vi "Check Status.vi"(8 "error in (no error)":errorcluster, 11 "Photon Counter SR400 in":refnum<class "Photon Counter SR400.lvclass">) -> (0 "error out":errorcluster, 1 "response":string caption="Status", 2 "Ready?":bool, 3 "Photon Counter SR400 out":refnum<class "Photon Counter SR400.lvclass">)   [LabVIEW 2012, in "Photon Counter SR400.lvclass"]
doc: "Checks if the instrument is powered on and updates its member data with the instrument's current status.\n\nNote: it's impossible to get the \"trigger frequency\" (one of the member data) from the instrument itself. Perhaps it shouldn't be part of the member data, but having it as member data makes it possible to give a counting time, which seems like a very important instrumental parameter. Therefore this VI tries to pull the trigger frequency off the existing member data, which won't work when first initialized. Don't know if there will be issues that arise because of that."
uses:
  Photon Counter SR400.lvclass
  Utility Classes/Readable/Readable.lvclass
  Photon Counter SR400.lvclass/Photon Counter SR400.ctl
  SR400/SR400.lvlib
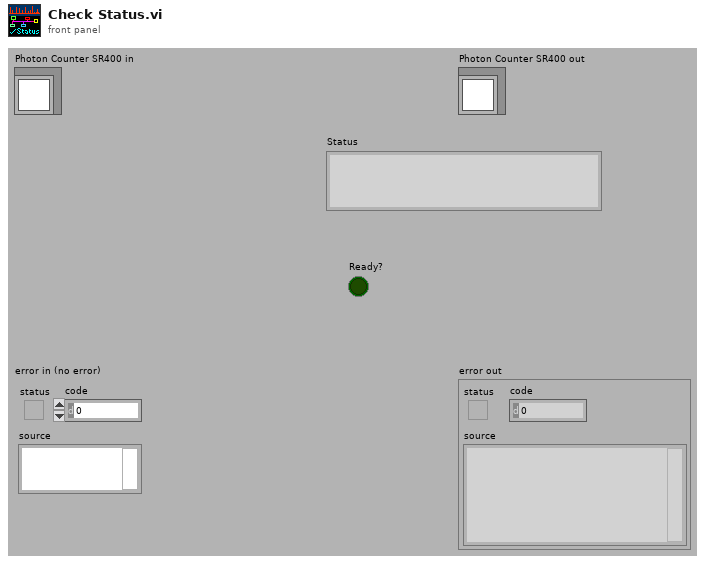
[diagram p1: front panel]
types:
  T1 = typedef "SR400.lvlib/Counter Mode.ctl" = enum16{"A,B For T Preset", "A-B For T Preset", "A+B For T Preset", "A For B Preset"}
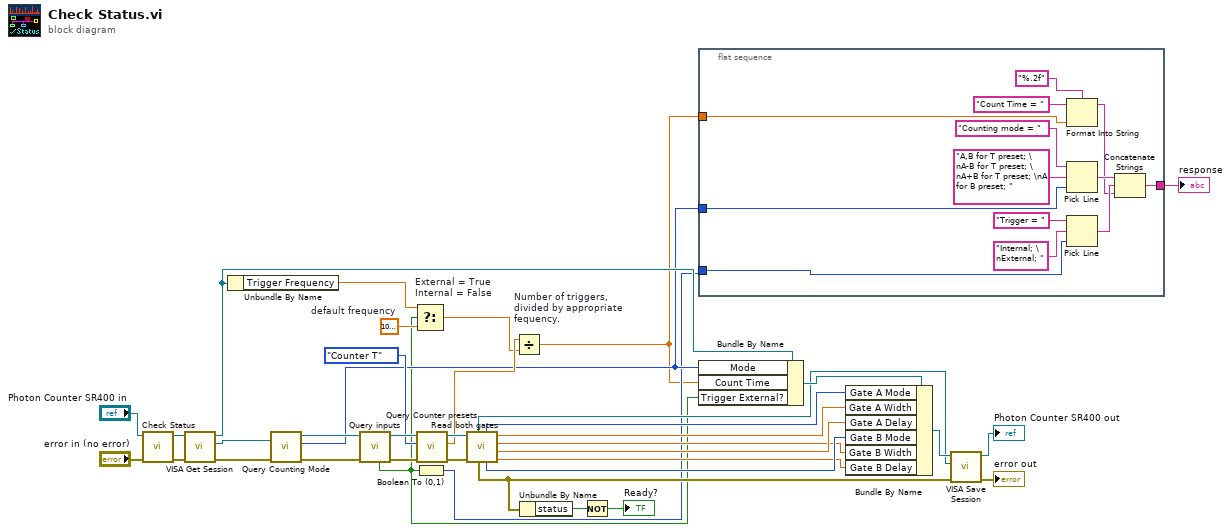
[diagram p0: block diagram]
diagram:
  w9 = dbl[unit] 10000000.0  # default frequency
  n1 = call-parent "Check Status.vi"("error in (no error)"="error in (no error)", "Instrument in"="Photon Counter SR400 in") -> ("error out"=w31:errorcluster, "Instrument out"=w33:refnum<class "Photon Counter SR400.lvclass">)  [unwired: 8 out]
  n2 = call-dynamic "VISA Get Session.vi"("error in (no error)"=w31, "Instrument.lvclass in"=w33) -> ("error out"=w11:errorcluster, "VISA Resource Name"=w1:refnum<visa-resource-name>, "Instrument.lvclass out"=w13:refnum<class "Photon Counter SR400.lvclass">)  [unwired: 7 out]
  n3 = Unbundle By Name(w13) -> ("Trigger Frequency"=w8:dbl[unit])
  n4 = call "Query Counting Mode.vi"("error in (no error)"=w11, "VISA resource name"=w1) -> ("error out"=w10:errorcluster, "output"=w5:T1, "VISA resource name out"=w12:refnum<visa-resource-name>)  [unwired: 7 out]
  n5 = call "Query inputs.vi"("error in (no error)"=w10, "VISA resource name"=w12) -> ("error out"=w25:errorcluster, "VISA resource name out"=w26:refnum<visa-resource-name>, "Externally-triggered?"=w4:bool)  [unwired: 7 out]
  n6 = Select "External = True\nInternal = False"(t=w8, s=w4, f=w9) -> (s? t:f=w6:dbl[unit])
  n7 = Boolean To (0,1)(Boolean=w4) -> (0, 1=w3:i16)
  n8 = call "Query Counter presets.vi"("error in (no error)"=w25, "Counter (Def: T)"=enum16{"Invalid", "Counter B", "Counter T"}."Counter T" ("i (0)"), "VISA resource name"=w26) -> ("error out"=w28:errorcluster, "Number of triggers"=w7:dbl, "VISA resource name out"=w29:refnum<visa-resource-name>)  [unwired: 6 out]
  n9 = call "Read both gates.vi"("error in (no error)"=w28, "VISA resource name"=w29) -> ("Gate B Delay"=w18:dbl[unit], "Gate A Delay"=w21:dbl[unit], "Gate B Width"=w19:dbl[unit], "Gate A Width"=w22:dbl[unit], "Current mode B"=w20:enum16{"CW", "Fixed", "Scan"}, "Current mode A"=w23:enum16{"CW", "Fixed", "Scan"}, "error out"=w15:errorcluster, "VISA resource name out"=w16:refnum<visa-resource-name>)  [unwired: 2 out]
  n10 = Divide "Number of triggers,\ndivided by appropriate\nfequency."(x=w7, y=w6) -> (x/y=w2:dbl[unit])
  n11 = Unbundle By Name(w15) -> ("status"=w14:bool)
  n12 = Not(x=w14) -> (.not. x?=→"Ready?":bool)
  n13 = flat-sequence {
    tunnel: [w46] -> w34
    tunnel: w5 -> [w48]
    tunnel: w3 -> [w43]
    tunnel: w2 -> [w40]
    frame #0 {
      n14 = Format Into String(format string="%.2f", initial string="Count Time = " ("string (\"\")"), w40) -> (resulting string=w39:string)  [unwired: 1 in, 1 out]
      n15 = Pick Line(string ("")="Counting mode = ", multi-line string="A,B for T preset; \nA-B for T preset; \nA+B for T preset; \nA for B preset; ", line index=w48) -> (output string=w47:string)
      n16 = Pick Line(string ("")="Trigger = ", multi-line string="Internal; \nExternal; ", line index=w43) -> (output string=w42:string)
      n17 = Concatenate Strings(w47, w42, w39) -> (w46:string)
    }
  }
  n18 = Bundle By Name(cluster=w13, "Mode"=w5, "Count Time"=w2, "Trigger External?"=w4) -> (w27:refnum<class "Photon Counter SR400.lvclass">)
  n19 = Bundle By Name(cluster=w27, "Gate A Mode"=w23, "Gate A Width"=w22, "Gate A Delay"=w21, "Gate B Mode"=w20, "Gate B Width"=w19, "Gate B Delay"=w18) -> (w17:refnum<class "Photon Counter SR400.lvclass">)
  n20 = call-dynamic "VISA Save Session.vi"("error in (no error)"=w15, "VISA Resource Name"=w16, "Instrument.lvclass in"=w17) -> ("error out"=→"error out":errorcluster, "Instrument.lvclass out"=→"Photon Counter SR400 out":refnum<class "Photon Counter SR400.lvclass">)  [unwired: 7 out]
  "response" <- w34
